vi "Change to Idle State.vi"(8 "error in (no error)":errorcluster, 11 "Test UI in":refnum<class "Test UI.lvclass">) -> (0 "error out":errorcluster, 3 "Test UI out":refnum<class "Test UI.lvclass">)   [LabVIEW 2024, in "Test UI.lvlib" / "Test UI.lvclass"]
uses:
  Test UI.lvclass
  Test UI.lvclass/Test UI.ctl
  Test States/Test State Messages/Go to Idle Msg/Go to Idle Msg.lvclass
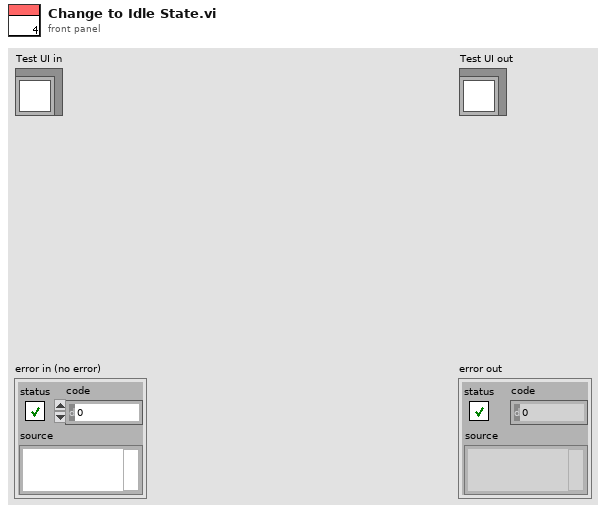
[diagram p1: front panel]
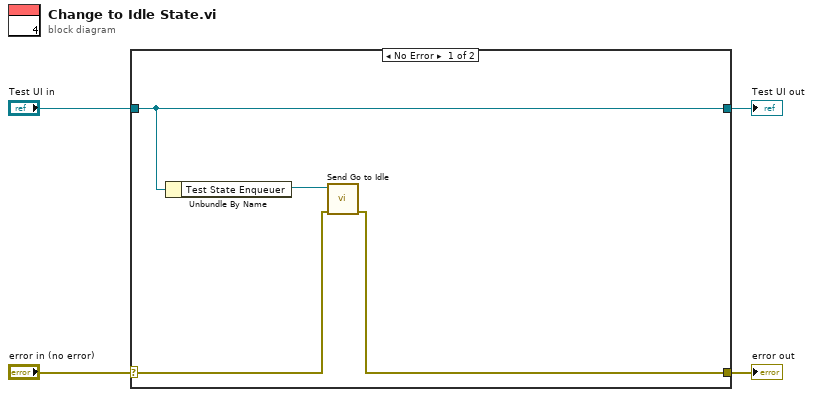
[diagram p0: block diagram]
diagram:
  n1 = case shown="No Error" "error in (no error)" {
    selector: "error in (no error)" -> [w6 w10]
    tunnel: [w5 w10] -> w3
    tunnel: [w8 w9] -> w1
    tunnel: "Test UI in" -> [w8 w9]
    frame No Error {
      n2 = Unbundle By Name(w8) -> ("Test State Enqueuer"=w7:refnum<class "Message Enqueuer.lvclass">)
      n3 = call "Send Go to Idle.vi"("error in (no error)"=w6, "Message Enqueuer"=w7) -> ("error out"=w5:errorcluster)  [unwired: 8 in, 1 out]
    }
    frame Error {
    }
  }
  "error out" <- w3
  "Test UI out" <- w1
